vi "GenerateDualFrequencyWaveform.vi"(7 "Phase (2pi unit)":dbl, 8 "Enum":enum16{"sinus", "triangle"}(ring)=enum."triangle", 9 "Freq US (Hz)":dbl=80000000.0, 10 "Harmonic":dbl=1.0, 11 "WaveDuration (us)":dbl=2e-05) -> (0 "High Frequency OUT":dbl=100000.0, 1 "Low Frequency OUT":dbl=100000.0, 2 "Waveforms":dbl[][](graph), 3 "OutPut Points":i32[](array[numeric]), 4 "Sample Frequency (Hz)":dbl, 5 "Freq CH2 (Hz)":dbl)   [LabVIEW 2015, in "ArbitraryFunctions.lvlib"]
uses:
  ArbitraryFunctions.lvlib
panel:
  out "N points":i32
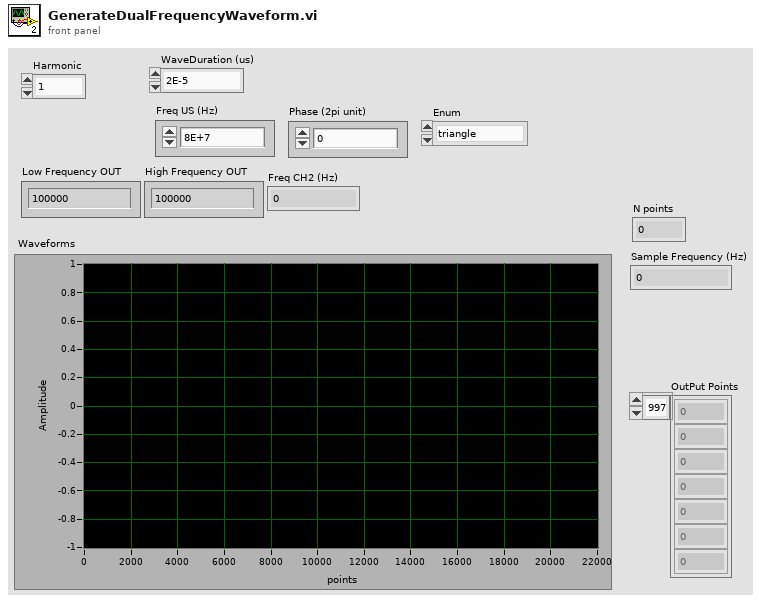
[diagram p1: front panel]
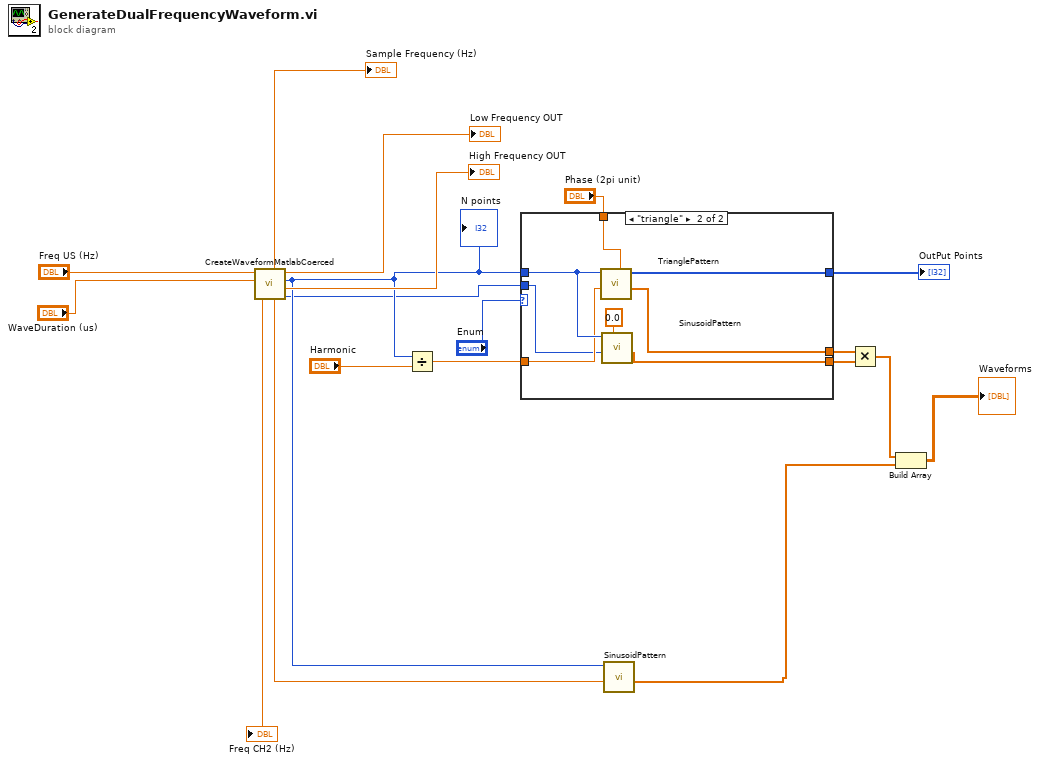
[diagram p0: block diagram]
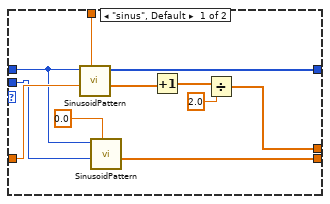
[diagram p2: hidden frame]
diagram:
  n1 = call "CreateWaveformMatlabCoerced.vi"("WaveDuration (us)"="WaveDuration (us)", "Freq US  (Hz)"="Freq US (Hz)") -> ("NCH1 high"=w3:i32, "Freq CH1  (Hz)"=→"High Frequency OUT":dbl, "Nlow"=w4:i32, "Freq Low"=→"Low Frequency OUT":dbl, "NCH2 high"=w11:dbl, "sampling frequency"=→"Sample Frequency (Hz)":dbl, "Freq CH2 (Hz)"=→"Freq CH2 (Hz)":dbl)  [unwired: 3 in]
  "N points" <- w4
  n2 = Divide(x=w4, y="Harmonic") -> (x/y=w14:dbl)
  n3 = case shown="\"triangle\"" "Enum" {
    tunnel: [w24 w36] -> w13
    tunnel: [w30 w35] -> w19
    tunnel: "Phase (2pi unit)" -> [w29 w37]
    tunnel: [w27 w38] -> w17
    tunnel: w14 -> [w22 w33]
    tunnel: w4 -> [w20 w34]
    tunnel: w3 -> [w21 w32]
    frame "sinus", Default {
      n4 = call "SinusoidPattern.vi"("Phase (2pi unit)"=w29, "Frequency Ratio"=w22, "N point"=w20) -> ("Unit Pattern"=w25:dbl[], "Points"=w27:i32[])  [unwired: 7 in]
      n5 = call "SinusoidPattern.vi"("Phase (2pi unit)"=0.0, "Frequency Ratio"=w21, "N point"=w20) -> ("Unit Pattern"=w30:dbl[])  [unwired: 7 in, 1 out]
      n6 = Increment(x=w25) -> (x+1=w23:dbl[])
      n7 = Divide(x=w23, y=2.0) -> (x/y=w24:dbl[])
    }
    frame "triangle" {
      n8 = call "TrianglePattern.vi"("Phase (2pi unit)"=w37, "Ratio"=w33, "N"=w34) -> ("vector"=w36:dbl[], "points"=w38:i32[])  [unwired: 7 in]
      n9 = call "SinusoidPattern.vi"("Phase (2pi unit)"=0.0, "Frequency Ratio"=w32, "N point"=w34) -> ("Unit Pattern"=w35:dbl[])  [unwired: 7 in, 1 out]
    }
  }
  "OutPut Points" <- w17
  n10 = call "SinusoidPattern.vi"("Frequency Ratio"=w11, "N point"=w4) -> ("Unit Pattern"=w15:dbl[])  [unwired: 8 in, 1 out]
  n11 = Multiply(x=w13, y=w19) -> (x*y=w2:dbl[])
  n12 = Build Array(w2, w15) -> (→"Waveforms":dbl[][])
